vi "Grab Target Info.vi"(8 "error in (no error)":errorcluster, 11 "Refnum in":refnum<k21>) -> (0 "error out":errorcluster, 2 "Network Module Information":T1 {"IP Mode" items=["Static"=1, "DHCP/Link-Local"=2, "Link-Local Only"=4, "DHCP Only"=8]}, 3 "Refnum out":refnum<k21>)   [LabVIEW 2013]
uses:
  types/MAX Sys Cfg Target Information.ctl
  <resource>/objmgr/nisysapi.rc
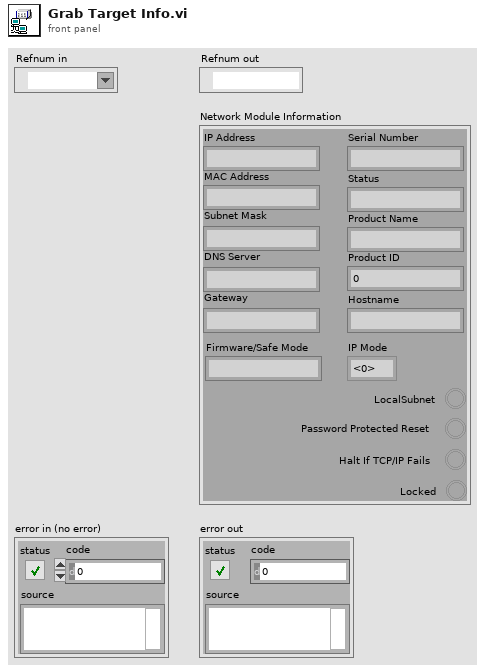
[diagram p1: front panel]
types:
  T1 = typedef "MAX Sys Cfg Target Information.ctl" = cluster{"MAC Address":string, "IP Address":string, "Status":string, "Product Name":string, "Hostname":string, "Firmware/Safe Mode":string, "Subnet Mask":string, "Gateway":string, "DNS Server":string, "Serial Number":string, "Product ID":u32, "Locked ":bool, "LocalSubnet":bool, "Halt If TCP/IP Fails":bool, "Password Protected Reset":bool, "IP Mode":i32}
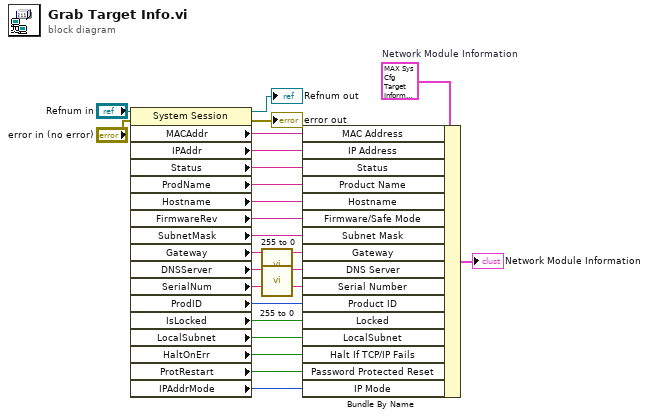
[diagram p0: block diagram]
diagram:
  w21 = T1 {"MAC Address"="", "IP Address"="", "Status"="", "Product Name"="", "Hostname"="", "Firmware/Safe Mode"="", "Subnet Mask"="", "Gateway"="", "DNS Server"="", "Serial Number"="", "Product ID"=0, "Locked "=FALSE, "LocalSubnet"=FALSE, "Halt If TCP/IP Fails"=FALSE, "Password Protected Reset"=FALSE, "IP Mode"=0}  # Network Module Information
  n1 = property class="System Session"(reference="Refnum in", error in="error in (no error)") -> (reference out=→"Refnum out":refnum<k21>, error out=→"error out":errorcluster, "MACAddr"=w3:string, "IPAddr"=w4:string, "Status"=w5:string, "ProdName"=w6:string, "Hostname"=w7:string, "FirmwareRev"=w8:string, "SubnetMask"=w18:string, "Gateway"=w9:string, "DNSServer"=w10:string, "SerialNum"=w11:string, "ProdID"=w12:i32, "IsLocked"=w13:bool, "LocalSubnet"=w14:bool, "HaltOnErr"=w15:bool, "ProtRestart"=w16:bool, "IPAddrMode"=w17:i32)
  n2 = call "255 to 0.vi"("255"=w9) -> ("0"=w24:string)  [unwired: 10 in]
  n3 = call "255 to 0.vi"("255"=w10) -> ("0"=w23:string)  [unwired: 10 in]
  n4 = Bundle By Name(cluster=w21, "MAC Address"=w3, "IP Address"=w4, "Status"=w5, "Product Name"=w6, "Hostname"=w7, "Firmware/Safe Mode"=w8, "Subnet Mask"=w18, "Gateway"=w24, "DNS Server"=w23, "Serial Number"=w11, "Product ID"=w12, "Locked"=w13, "LocalSubnet"=w14, "Halt If TCP/IP Fails"=w15, "Password Protected Reset"=w16, "IP Mode"=w17) -> (→"Network Module Information":T1)
